vi "Table RW.vi"(3 "Error In":errorcluster, 5 "Table In":T1[](array[typedef])) -> (0 "Error Out":errorcluster, 1 "Number of param":i32, 2 "List Out":string[][](array[string]))   [LabVIEW 2018]
uses:
  GC-MSMSDevlopment/Type/_RT Configuration 2.ctl
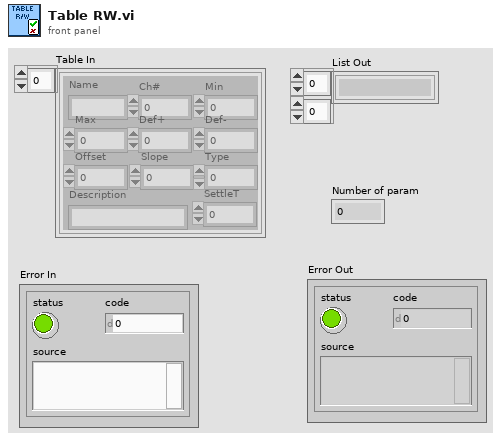
[diagram p1: front panel]
types:
  T1 = typedef "_RT Configuration 2.ctl" = cluster{"Name":string, "Ch#":u8, "Min":dbl, "Max":dbl, "Def+":dbl, "Def-":dbl, "Offset":dbl, "Slope":dbl, "Type":u8, "Description":string, "SettleT":dbl}
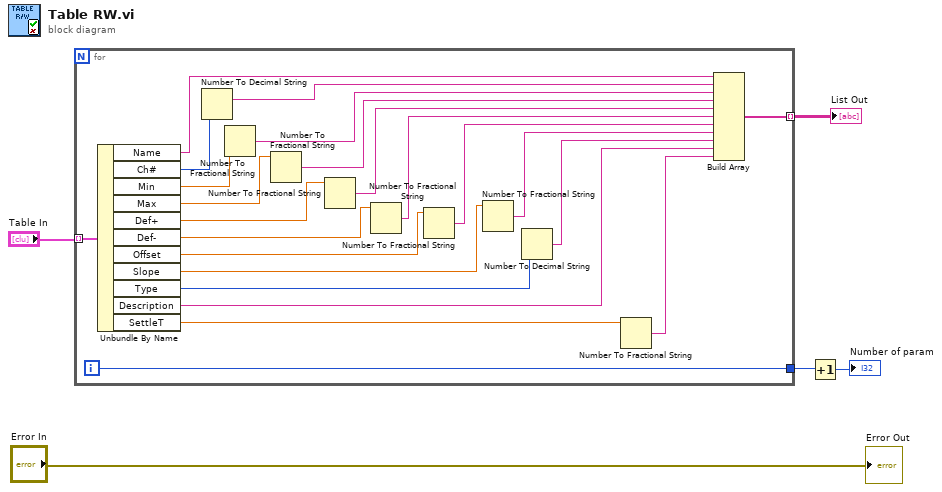
[diagram p0: block diagram]
diagram:
  n1 = for {
    tunnel: [w28] -> w5 mode=indexing
    tunnel: "Table In" -> [w24] mode=indexing
    tunnel: [w6] -> w3
    i -> [w6]
    n2 = Unbundle By Name(w24) -> ("Name"=w23:string, "Ch#"=w22:u8, "Min"=w21:dbl, "Max"=w20:dbl, "Def+"=w19:dbl, "Def-"=w17:dbl, "Offset"=w15:dbl, "Slope"=w13:dbl, "Type"=w11:u8, "Description"=w9:string, "SettleT"=w8:dbl)
    n3 = Number To Decimal String(number=w22) -> (decimal integer string=w27:string)  [unwired: 1 in]
    n4 = Number To Fractional String(number=w21) -> (F-format string=w26:string)  [unwired: 1 in, 2 out]
    n5 = Number To Fractional String(number=w20) -> (F-format string=w25:string)  [unwired: 1 in, 2 out]
    n6 = Number To Fractional String(number=w19) -> (F-format string=w18:string)  [unwired: 1 in, 2 out]
    n7 = Number To Fractional String(number=w17) -> (F-format string=w16:string)  [unwired: 1 in, 2 out]
    n8 = Number To Fractional String(number=w15) -> (F-format string=w14:string)  [unwired: 1 in, 2 out]
    n9 = Number To Fractional String(number=w13) -> (F-format string=w12:string)  [unwired: 1 in, 2 out]
    n10 = Number To Decimal String(number=w11) -> (decimal integer string=w10:string)  [unwired: 1 in]
    n11 = Number To Fractional String(number=w8) -> (F-format string=w7:string)  [unwired: 1 in, 2 out]
    n12 = Build Array(w23, w27, w26, w25, w18, w16, w14, w12, w10, w9, w7) -> (w28:string[])
  }
  "List Out" <- w5
  n13 = Increment(x=w3) -> (x+1=→"Number of param":i32)
  "Error Out" <- "Error In"
